vi "neutral_PixelFly_testVI.vi"() -> ()   [LabVIEW 2016]
uses:
  Controls/PixelFly/PixelFly Status Indicator.ctl
  Controls/PixelFly/PixelFly Buffer Status.ctl
  Controls/PixelFly/PixelFly_Control.ctl
  Controls/PixelFly/Acquisition Settings.ctl
  Controls/PixelFly/Bit_Depth_Enum.ctl
panel:
  out "Intensity Graph":dbl[][](graph)
  in  "stop":bool
  in  "PixelFly Control":T1={"Acquitsition Settings"={"Buffer number"=0, "Size (Bytes)"=5242880, "initialized array"=array2048x1280[2621440 elements], "X Bin"=1, "Y Bin"=1, "Board Handle"=16520, "Picture parameters"={"ccdxsize"=1280, "ccdy"=1024, "pictx"=1280, "picty"=2048, "bitspixel"=12}, "Buffer Out"=[]}, "Initialization"={"Exposure mode"=1, "exp time"=150, "exp level"=1, "gain"=0, "boardid in"=0, "offset"=0, "V bin"=0, "H bin"=0, "trigger"=FALSE, "Bit depth"=1}} {"Initialization"."Bit depth" items=["8", "12"]; "Initialization"."H bin" items=["1", "2"]; "Initialization"."V bin" items=["1", "2"]; "Initialization"."boardid in" min=0 max=3 step=1; "Initialization"."gain" items=["Low (X1)", "High (X2)"]; "Initialization"."exp level" min=0 max=255 step=1; "Initialization"."exp time" min=1 max=10000; "Initialization"."Exposure mode" items=["Asynch shutter", "Double shot", "Video mode", "Auto exposure"]}
  out "error out":errorcluster
  in  "error in":errorcluster
  out "Buffer status":T4
  out "PixelFly Status":T5={"Board Parameters"={"Type"=65, "Number"=1, "Initialized"=TRUE, "Running"=FALSE, "Lost head"=FALSE, "CCD X size"=1280, "CCD Y size"=1024, "Mode"=16, "Exposure time"=2500, "Exposure level"=100, "Horizontal bin"=0, "Vertical bin"=0, "Reg W"=FALSE, "Gain"=0, "Pixel depth"=12, "Bit Shift"=0, "Offset"=0, "Last exposure"=1000, "Double "=TRUE, "Light meter"=FALSE, "Color"=FALSE, "Open count"=2284934248, "Active buffer"=TRUE, "Next Buffer"=TRUE}, "CCD temp"=44} {"CCD temp" scale=0.0..100.0; "Board Parameters"."Vertical bin" items=["1", "2"]; "Board Parameters"."Horizontal bin" items=["1", "2"]}
  # "Status flags"
  # "Buffer errors"
  # "Memory usage"
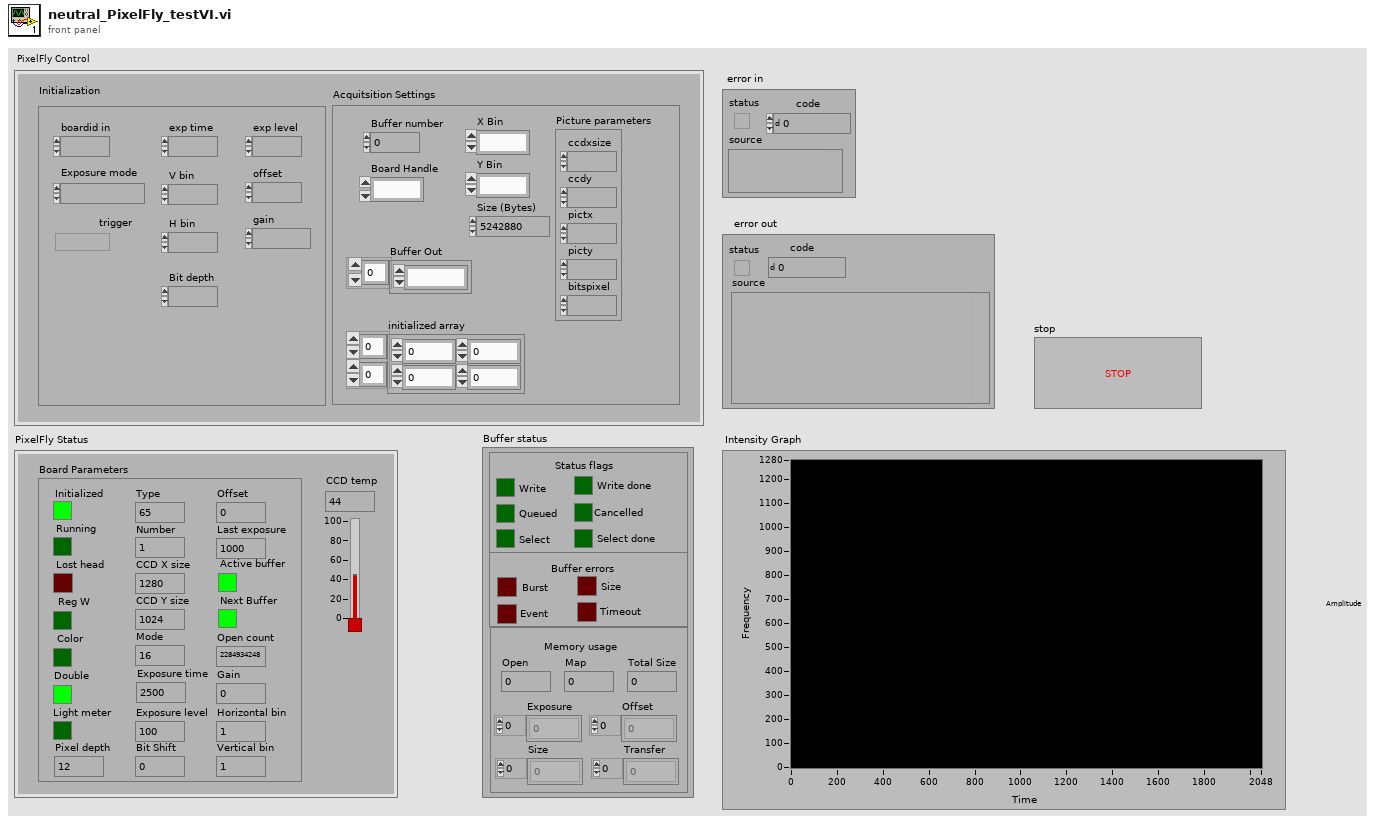
[diagram p1: front panel]
types:
  T1 = typedef "PixelFly_Control.ctl" = cluster{"Acquitsition Settings":T2, "Initialization":cluster{"Exposure mode":u16, "exp time":i32, "exp level":i32, "gain":i32, "boardid in":i32, "offset":i32, "V bin":i32, "H bin":i32, "trigger":bool, "Bit depth":T3}}
  T2 = typedef "Acquisition Settings.ctl" = cluster{"Buffer number":i32, "Size (Bytes)":i32, "initialized array":u16[][], "X Bin":i32, "Y Bin":i32, "Board Handle":u32, "Picture parameters":cluster{"ccdxsize":i32, "ccdy":i32, "pictx":i32, "picty":i32, "bitspixel":i32}, "Buffer Out":u16[]}
  T3 = typedef "Bit_Depth_Enum.ctl" = i32
  T4 = typedef "PixelFly Buffer Status.ctl" = cluster{"Write":bool, "Write done":bool, "Queued":bool, "Cancelled":bool, "Select":bool, "Select done":bool, "Burst":bool, "Size":bool, "Event":bool, "Timeout":bool, "Open":i32, "Map":i32, "Exposure":i32[], "Offset":i32[], "Size":i32[], "Transfer":i32[], "Total Size":i32}
  T5 = typedef "PixelFly Status Indicator.ctl" = cluster{"Board Parameters":cluster{"Type":u32, "Number":u32, "Initialized":bool, "Running":bool, "Lost head":bool, "CCD X size":u32, "CCD Y size":u32, "Mode":u32, "Exposure time":u32, "Exposure level":u32, "Horizontal bin":u32, "Vertical bin":u32, "Reg W":bool, "Gain":u32, "Pixel depth":i32, "Bit Shift":u32, "Offset":u32, "Last exposure":u32, "Double ":bool, "Light meter":bool, "Color":bool, "Open count":u32, "Active buffer":bool, "Next Buffer":bool}, "CCD temp":i32}
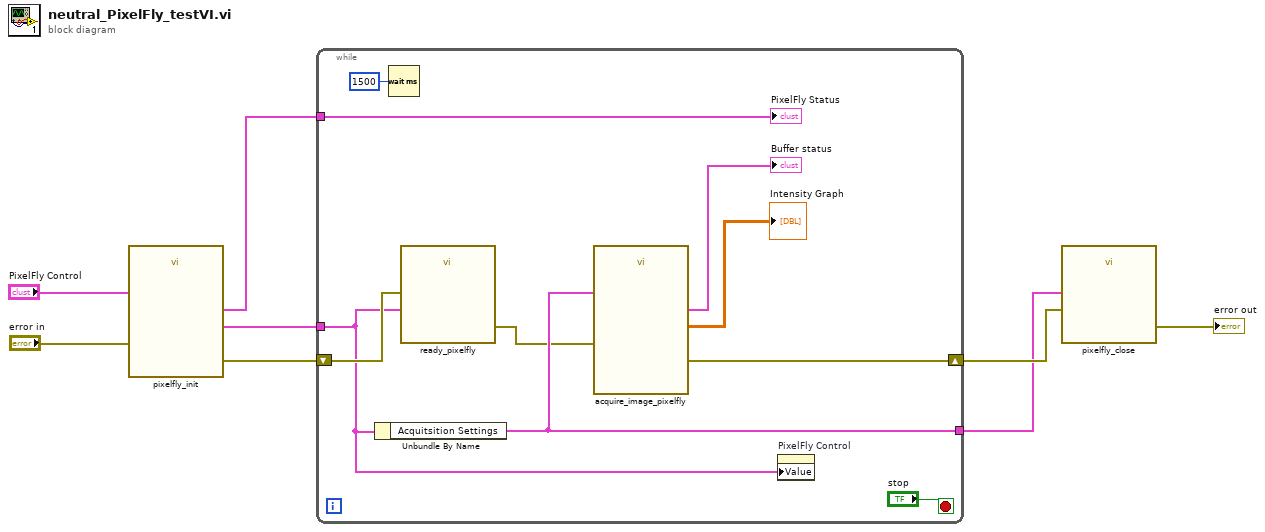
[diagram p0: block diagram]
diagram:
  n1 = call "pixelfly_init.vi"("error in (no error)"="error in", "PixelFly Controls"="PixelFly Control") -> ("error out"=w2:errorcluster, "PixelFly Status"=w7:T5, "PixelFly Controls Out"=w1:T1)  [unwired: 1 in]
  n2 = while {
    tunnel: w7 -> [w17]
    tunnel: [w15] -> w3
    tunnel: w1 -> [w12]
    shift-right: [w18] -> w8
    shift-left: w2 -> [w14]
    stop <- "stop" stop-if-true
    n3 = Unbundle By Name(w12) -> ("Acquitsition Settings"=w15:T2)
    n4 = Wait (ms)(milliseconds to wait=u32 1500) -> ()  [unwired: 1 out]
    n5 = call "ready_pixelfly.vi"("error in"=w14, "PixelFly Controls"=w12) -> ("error out"=w13:errorcluster)  [unwired: 3 in]
    n6 = call "acquire_image_pixelfly.vi"("error in"=w13, "Acquitsition Settings"=w15) -> ("error out"=w18:errorcluster, "Buffer status"=→"Buffer status":T4, "Output array"=→"Intensity Graph":dbl[][])  [unwired: 1 in]
    n7 = property on="PixelFly Control" class="Clust (strict)"("Value"=w12) -> ()  [unwired: 2 in, 2 out]
    "PixelFly Status" <- w17
  }
  n8 = call "pixelfly_close.vi"("error in (no error)"=w8, "Acquitsition Settings"=w3) -> ("error out"=→"error out":errorcluster)  [unwired: 2 in]
